vi "Get Checked Elements.vi"(9 "index":i32=6, 10 "Checks":bool[](array[boolean]), 11 "tokens":cluster{"token type":T2, T3}[](array[cluster])) -> (3 "Found Token Info":T1(array[cluster]))   [LabVIEW 2019]
doc: "Search the root level of the tokenized JSON identifying fields with the names of interest. Outputs contain strings, but are not necessarily in the requested order."
uses:
  <vilib>/MultiError/TokenizeJSON/JSON Token Values.ctl
  <vilib>/MultiError/Errors Cluster Multiple Errors/JSON Token Descriptor.ctl
  <vilib>/MultiError/TokenizeJSON/JSON Raw Token Values.ctl
  <vilib>/MultiError/TokenizeJSON/Multi Error Cluster.lvlib
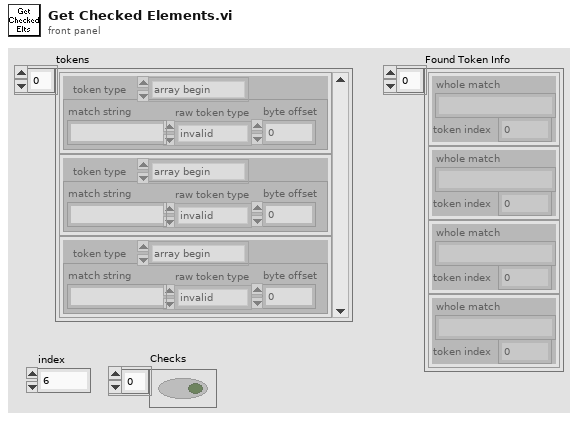
[diagram p1: front panel]
types:
  T1 = cluster{"whole match":string, "token index":i32}[]
  T2 = typedef "Multi Error Cluster.lvlib/JSON Token Values.ctl" = enum32{"array begin", "array end", "object begin", "object end", "value", "invalid", "name"}
  T3 = typedef "Multi Error Cluster.lvlib/JSON Token Descriptor.ctl" = cluster{"match string":string, "raw token type":T4, "byte offset ":i32}
  T4 = typedef "Multi Error Cluster.lvlib/JSON Raw Token Values.ctl" = enum32{"{", "}", "[", "]", ",", ":", "\"", "number", "string", "true", "false", "null", "invalid"}
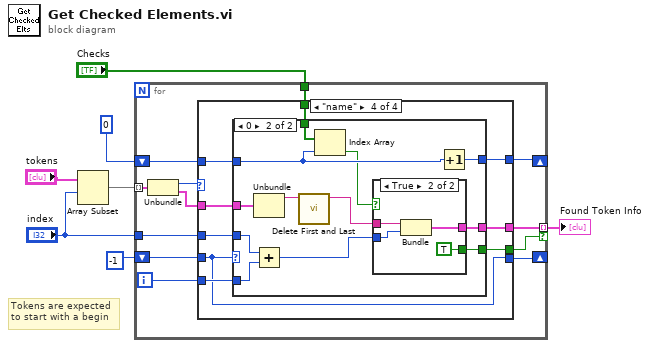
[diagram p0: block diagram]
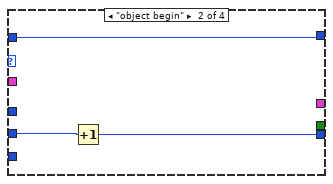
[diagram p3: hidden frame]
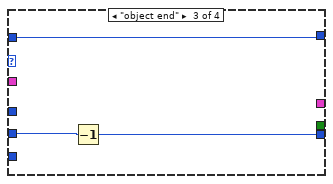
[diagram p4: hidden frame]
diagram:
  # "Tokens are expected\nto start with a begin"
  n1 = Array Subset(array="tokens", index="index") -> (w2:cluster{"token type":T2, T3}[])  [unwired: 1 in]
  n2 = for {
    tunnel: w2 -> [w19] mode=indexing
    tunnel: "Checks" -> [w18]
    tunnel: [w16] -> w6 mode=indexing if=w15
    shift-right: [w13] -> _
    shift-left: -1 -> [w14]
    shift-right: [w9] -> _
    shift-left: 0 -> [w10]
    tunnel: "index" -> [w8]
    i -> [w17]
    n3 = Unbundle(w19) -> ("token type"=w12:T2, w11:T3)
    n4 = case shown="\"name\"" w12 {
      tunnel: w11 -> [_ _ _ w36]
      tunnel: w18 -> [_ _ _ w35]
      tunnel: w17 -> [_ _ _ w34]
      tunnel: [_ _ _ w33] -> w16
      tunnel: [_ _ _ w32] -> w15
      tunnel: w14 -> [w21 w24 w27 w31]
      tunnel: [w21 w23 w26 w31] -> w13
      tunnel: w10 -> [w20 w22 w25 w30]
      tunnel: [w20 w22 w25 w29] -> w9
      tunnel: w8 -> [_ _ _ w28]
      frame Default {
      }
      frame "object begin" {
        n5 = Increment(x=w24) -> (x+1=w23:i32)
      }
      frame "object end" {
        n6 = Decrement(x=w27) -> (x-1=w26:i32)
      }
      frame "name" {
        n7 = case shown="0" w31 {
          tunnel: w36 -> [_ w49]
          tunnel: w35 -> [_ w43]
          tunnel: w34 -> [_ w39]
          tunnel: [_ w48] -> w33
          tunnel: [_ w47] -> w32
          tunnel: w30 -> [w37 w42]
          tunnel: [w37 w44] -> w29
          tunnel: w28 -> [_ w38]
          frame Default {
          }
          frame 0 {
            n8 = Unbundle(w49) -> ("match string"=w46:string)  [unwired: 2 out]
            n9 = Add(x=w38, y=w39) -> (x+y=w40:i32)
            n10 = call <vilib>:"Delete First and Last.vi"("string in"=w46) -> ("string subset"=w45:string)  [unwired: 10 in]
            n11 = Index Array(array=w43, index=w42) -> (element=w41:bool)
            n12 = case shown="True" w41 {
              tunnel: w45 -> [_ w53]
              tunnel: w40 -> [_ w50]
              tunnel: [_ w52] -> w48
              tunnel: [_ TRUE] -> w47
              frame False {
              }
              frame True {
                n13 = Bundle("string subset"=w53, w50) -> (w52:cluster{"string subset":string, i32})  [unwired: 1 in]
              }
            }
            n14 = Increment(x=w42) -> (x+1=w44:i32)
          }
        }
      }
    }
  }
  "Found Token Info" <- w6
